vi "Full Force Test SAA.vi"(8 "error in (no error)":errorcluster, 10 "Model in":refnum<class "Model.lvclass">, 11 "Test Actuator State in":refnum<class "Test Actuator State.lvclass">) -> (0 "error out":errorcluster, 1 "Pass":bool, 2 "Model out":refnum<class "Model.lvclass">, 3 "Test Actuator State out":refnum<class "Test Actuator State.lvclass">)   [LabVIEW 2016, in "Test Actuator State.lvclass"]
uses:
  Test Actuator State.lvclass
  Model/Model/Model.lvclass
  Model/Model/Model.lvclass/Model.ctl
  Typedefs/ActuatorSetPoints.ctl
  <vilib>/Platform/TimedLoop/XDataNode/timing_clust.ctl
  <vilib>/Platform/TimedLoop/XDataNode/nitl_modes.ctl
  <vilib>/Platform/TimedLoop/XDataNode/wakeup.ctl
  <vilib>/platform/TimedLoop/XDataNode/XDataNode.xnode
  Typedefs/FAMT Typedefs.lvlib
  <vilib>/Platform/TimedLoop/XDataNode/XDNodeRunTimeDep.lvlib
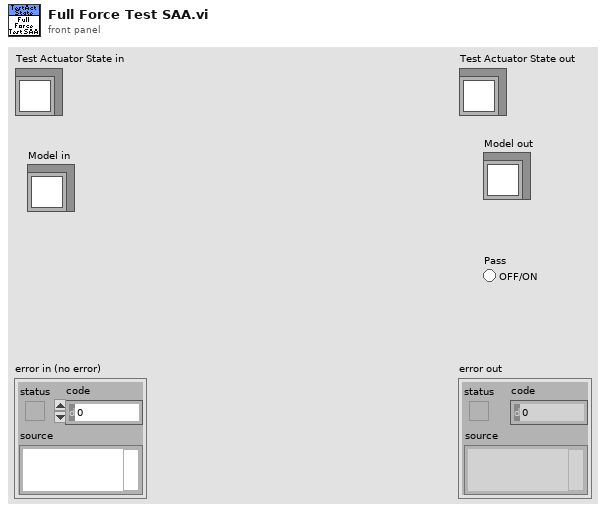
[diagram p1: front panel]
types:
  T1 = typedef "FAMT Typedefs.lvlib/FullForceScanSettings.ctl" = cluster{"Force Tolerance (N)":dbl, "DAA Force Set Points":T2[], "Process Time (s)":dbl, "Sample Time (s)":dbl, "Max Moment (NM)":dbl, "SAA Force Set Points":T2[]}
  T2 = typedef "FAMT Typedefs.lvlib/ForcePair.ctl" = cluster{"Axial Force":dbl, "Lateral Force":dbl}
  T3 = typedef "FAMT Typedefs.lvlib/ActuatorSetPoints.ctl" = cluster{"Axial Force":dbl, "Lateral Force":dbl, "FC1 Force":dbl, "FC2 Force":dbl}
  T4 = typedef "XDNodeRunTimeDep.lvlib/timing_clust.ctl" = cluster{"Expected End [f-1]":u64, "Actual End [f-1]":u64, "Finished Late? [f-1]":bool, "Expected End [i-1]":u64, "Actual End [i-1]":u64, "Finished Late? [i-1]":bool, "Expected Start [i]":u64, "Actual Start [i]":u64, "Expected Start [f]":u64, "Actual Start [f]":u64, "Source Name":string, "Structure Name":string, "Period":i64, "Deadline":i64, "Offset":i64, "Start":i64, "Priority":i32, "Timeout":i32, "Mode":T5, "Wakeup Reason":T6, "Error":errorcluster, "Source Type":string, "Secondary Source Type":string, "Global End Time":u64, "Global Start Time":u64, "Frame Duration":u64, "Iteration Duration":u64, "Assigned CPU":i32, "I/O Scan Engine Mode":u32}
  T5 = typedef "XDNodeRunTimeDep.lvlib/nitl_modes.ctl" = enum32{"No Change", "Process missed periods, maintain original phase", "Discard missed periods, maintain original phase", "Process missed periods, ignore original phase", "Discard missed periods, ignore original phase"}
  T6 = typedef "XDNodeRunTimeDep.lvlib/wakeup.ctl" = enum32{"Normal", "Aborted", "Asynchronous wakeup", "Timing source error", "Timed loop error", "Timeout"}
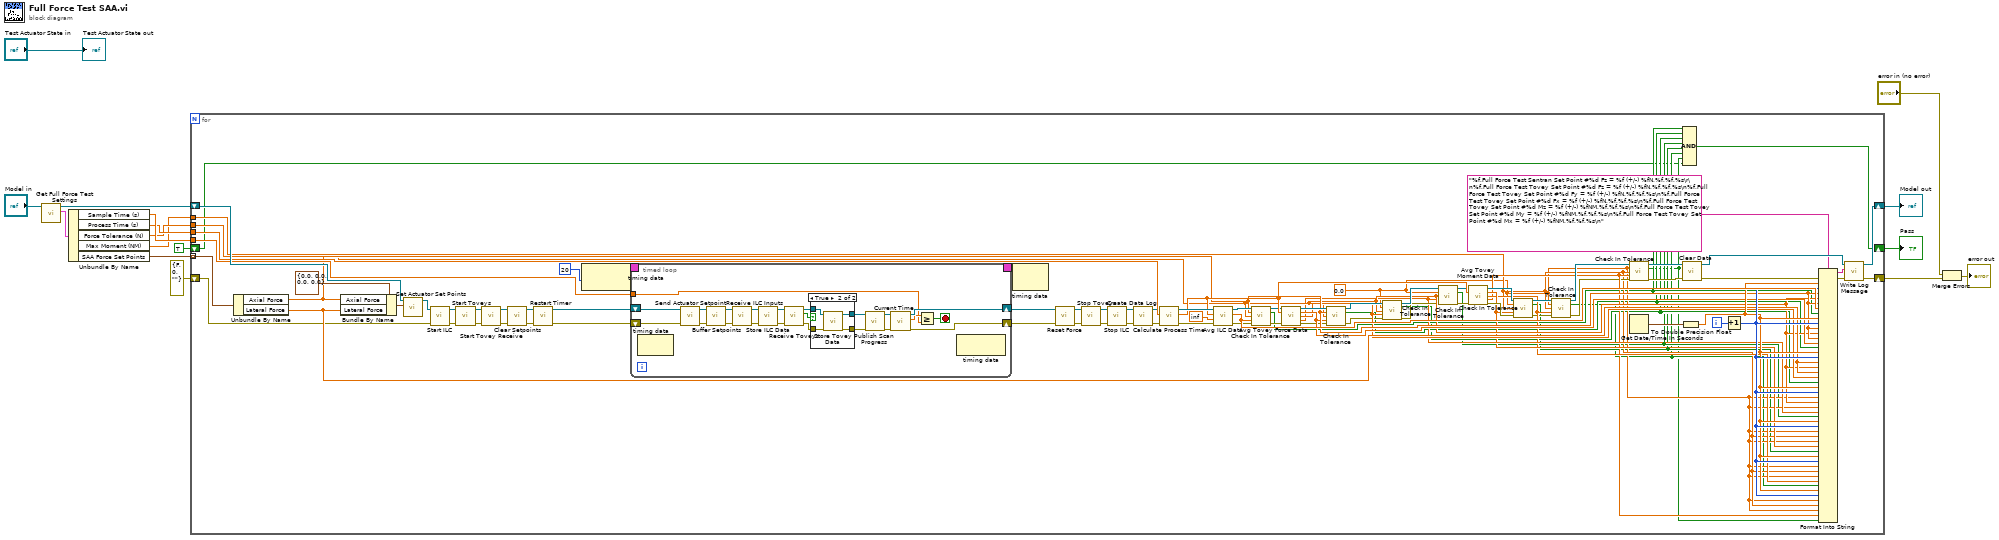
[diagram p0: block diagram]
diagram:
  n1 = call "Get Full Force Test Settings.vi"("Model in"="Model in") -> ("Full Force Test Settings"=w5:T1, "Model out"=w15:refnum<class "Model.lvclass">)  [unwired: 9 in]
  n2 = Unbundle By Name(w5) -> ("Sample Time (s)"=w14:dbl, "Process Time (s)"=w13:dbl, "Force Tolerance (N)"=w12:dbl, "Max Moment (NM)"=w7:dbl, "SAA Force Set Points"=w4:T2[])
  n3 = for {
    tunnel: w4 -> [w94] mode=indexing
    shift-right: [w99] -> w9
    shift-left: w15 -> [w102]
    tunnel: w14 -> [w101]
    tunnel: w13 -> [w89]
    tunnel: w12 -> [w73]
    shift-right: [w90] -> w8
    shift-left: errorcluster {"status"=FALSE, "code"=0, "source"=""} ("error out") -> [w40]
    tunnel: w7 -> [w55]
    shift-right: [w21] -> w1
    shift-left: TRUE -> [w22]
    i -> [w96]
    w54 = 0.0
    n4 = Unbundle By Name(w94) -> ("Axial Force"=w79:dbl, "Lateral Force"=w76:dbl)
    n5 = Bundle By Name(cluster=T3 {"Axial Force"=0.0, "Lateral Force"=0.0, "FC1 Force"=0.0, "FC2 Force"=0.0} ("Actuator Set Points"), "Axial Force"=w79, "Lateral Force"=w76) -> (w95:T3)
    n6 = call "Set Actuator Set Points.vi"("Actuator Set Points"=w95, "Model in"=w102) -> ("Model out"=w41:refnum<class "Model.lvclass">)  [unwired: 9 in]
    n7 = call "Start ILC.vi"("error in (no error)"=w40, "Model in"=w41) -> ("error out"=w39:errorcluster, "Model out"=w38:refnum<class "Model.lvclass">)  [unwired: 8 in]
    n8 = call "Start Toveys.vi"("error in (no error)"=w39, "Model in"=w38) -> ("error out"=w43:errorcluster, "Model out"=w45:refnum<class "Model.lvclass">)  [unwired: 8 in]
    n9 = call "Start Tovey Receive.vi"("error in (no error)"=w43, "Model in"=w45) -> ("error out"=w17:errorcluster, "Model out"=w20:refnum<class "Model.lvclass">)  [unwired: 8 in]
    n10 = call "Clear Setpoints.vi"("error in (no error)"=w17, "Model in"=w20) -> ("error out"=w18:errorcluster, "Model out"=w19:refnum<class "Model.lvclass">)  [unwired: 8 in]
    n11 = call "Restart Timer.vi"("error in (no error)"=w18, "Model in"=w19) -> ("error out"=w42:errorcluster, "Model out"=w44:refnum<class "Model.lvclass">)  [unwired: 8 in]
    n12 = node-c288(i64 20 ("Period")) -> (w50:T4)
    n13 = timed-loop {
      shift-right: [w123] -> w30
      shift-left: w44 -> [w125]
      shift-right: [w122] -> w33
      shift-left: w42 -> [w124]
      tunnel: w101 -> [w120]
      timing: w50 -> [_]
      timing-out: [_] -> w49
      stop <- w119 stop-if-true
      n14 = node-c288() -> ()  [unwired: 1 in, 1 out]
      n15 = call "Send Actuator Setpoint.vi"("error in (no error)"=w124, "Model in"=w125) -> ("error out"=w105:errorcluster, "Model out"=w107:refnum<class "Model.lvclass">)  [unwired: 8 in]
      n16 = call "Buffer Setpoints.vi"("error in (no error)"=w105, "Model in"=w107) -> ("error out"=w104:errorcluster, "Model out"=w106:refnum<class "Model.lvclass">)  [unwired: 8 in]
      n17 = call "Receive ILC Inputs.vi"("error in (no error)"=w104, "Model in"=w106) -> ("error out"=w108:errorcluster, "Model out"=w109:refnum<class "Model.lvclass">)  [unwired: 8 in]
      n18 = call "Store ILC Data.vi"("error in (no error)"=w108, "Model in"=w109) -> ("error out"=w117:errorcluster, "Model out"=w118:refnum<class "Model.lvclass">)  [unwired: 8 in]
      n19 = call "Receive Toveys.vi"("error in (no error)"=w117, "Model in"=w118) -> ("error out"=w115:errorcluster, "Data Received"=w114:bool, "Model out"=w116:refnum<class "Model.lvclass">)  [unwired: 7 in]
      n20 = case shown="True" w114 {
        tunnel: w116 -> [w129 w133]
        tunnel: w115 -> [w128 w132]
        tunnel: [w128 w131] -> w110
        tunnel: [w129 w130] -> w113
        frame False {
        }
        frame True {
          n21 = call "Store Tovey Data.vi"("error in (no error)"=w132, "Model in"=w133) -> ("error out"=w131:errorcluster, "Model out"=w130:refnum<class "Model.lvclass">)  [unwired: 8 in]
        }
      }
      n22 = call "Publish Scan Progress.vi"("error in (no error)"=w110, "Model in"=w113) -> ("error out"=w111:errorcluster, "Model out"=w112:refnum<class "Model.lvclass">)  [unwired: 8 in]
      n23 = call "Current Time.vi"("error in (no error)"=w111, "Model in"=w112) -> ("error out"=w122:errorcluster, "Time"=w121:dbl, "Model out"=w123:refnum<class "Model.lvclass">)  [unwired: 7 in]
      n24 = Greater Or Equal?(x=w121, y=w120) -> (x >= y?=w119:bool)
      n25 = node-c288() -> ()  [unwired: 1 in, 1 out]
    }
    n26 = node-c288(w49) -> ()  [unwired: 1 out]
    n27 = call "Reset Force.vi"("error in (no error)"=w33, "Model in"=w30) -> ("error out"=w32:errorcluster, "Model out"=w31:refnum<class "Model.lvclass">)  [unwired: 8 in]
    n28 = call "Stop Toveys.vi"("error in (no error)"=w32, "Model in"=w31) -> ("error out"=w37:errorcluster, "Model out"=w36:refnum<class "Model.lvclass">)  [unwired: 8 in]
    n29 = call "Stop ILC.vi"("error in (no error)"=w37, "Model in"=w36) -> ("error out"=w34:errorcluster, "Model out"=w35:refnum<class "Model.lvclass">)  [unwired: 8 in]
    n30 = call "Create Data Log.vi"("error in (no error)"=w34, "Model in"=w35) -> ("error out"=w46:errorcluster, "Model out"=w47:refnum<class "Model.lvclass">)  [unwired: 8 in]
    n31 = call "Calculate Process Time.vi"("error in (no error)"=w46, "Seconds"=w89, "Model in"=w47) -> ("error out"=w87:errorcluster, "Time"=w86:dbl, "Model out"=w88:refnum<class "Model.lvclass">)  [unwired: 6 in]
    n32 = call "Avg ILC Data.vi"("error in (no error)"=w87, "Before This Time"=inf, "After This Time"=w86, "Model in"=w88) -> ("error out"=w83:errorcluster, "Fz"=w84:dbl, "Model out"=w85:refnum<class "Model.lvclass">)  [unwired: 4 in, 1 out]
    n33 = call "Check In Tolerance.vi"("Model in"=w85, "Expected"=w79, "Tolerance"=w73, "Actual"=w84, "error in (no error)"=w83) -> ("Model out"=w53:refnum<class "Model.lvclass">, "Pass"=w29:bool, "error out"=w52:errorcluster)  [unwired: 8 in]
    n34 = call "Avg Tovey Force Data.vi"("Model in"=w53, "After This Time"=w86, "error in (no error)"=w52) -> ("Model out"=w80:refnum<class "Model.lvclass">, "Fz"=w78:dbl, "Fy"=w75:dbl, "Fx"=w65:dbl, "error out"=w72:errorcluster)  [unwired: 8 in]
    n35 = call "Check In Tolerance.vi"("Model in"=w80, "Expected"=w79, "Tolerance"=w73, "Actual"=w78, "error in (no error)"=w72) -> ("Model out"=w77:refnum<class "Model.lvclass">, "Pass"=w28:bool, "error out"=w71:errorcluster)  [unwired: 8 in]
    n36 = call "Check In Tolerance.vi"("Model in"=w77, "Expected"=w54, "Tolerance"=w73, "Actual"=w75, "error in (no error)"=w71) -> ("Model out"=w74:refnum<class "Model.lvclass">, "Pass"=w27:bool, "error out"=w70:errorcluster)  [unwired: 8 in]
    n37 = call "Check In Tolerance.vi"("Model in"=w74, "Expected"=w54, "Tolerance"=w73, "Actual"=w65, "error in (no error)"=w70) -> ("Model out"=w68:refnum<class "Model.lvclass">, "Pass"=w26:bool, "error out"=w69:errorcluster)  [unwired: 8 in]
    n38 = call "Avg Tovey Moment Data.vi"("Model in"=w68, "After This Time"=w86, "error in (no error)"=w69) -> ("Model out"=w67:refnum<class "Model.lvclass">, "Mz"=w64:dbl, "My"=w61:dbl, "Mx"=w60:dbl, "error out"=w66:errorcluster)  [unwired: 8 in]
    n39 = call "Check In Tolerance.vi"("Model in"=w67, "Expected"=w54, "Tolerance"=w55, "Actual"=w64, "error in (no error)"=w66) -> ("Model out"=w63:refnum<class "Model.lvclass">, "Pass"=w25:bool, "error out"=w58:errorcluster)  [unwired: 8 in]
    n40 = call "Check In Tolerance.vi"("Model in"=w63, "Expected"=w54, "Tolerance"=w55, "Actual"=w61, "error in (no error)"=w58) -> ("Model out"=w62:refnum<class "Model.lvclass">, "Pass"=w24:bool, "error out"=w57:errorcluster)  [unwired: 8 in]
    n41 = call "Check In Tolerance.vi"("Model in"=w62, "Expected"=w54, "Tolerance"=w55, "Actual"=w60, "error in (no error)"=w57) -> ("Model out"=w59:refnum<class "Model.lvclass">, "Pass"=w23:bool, "error out"=w56:errorcluster)  [unwired: 8 in]
    n42 = Get Date/Time In Seconds() -> (seconds since 1Jan1904=w97:timestamp)
    n43 = To Double Precision Float(number=w97) -> (double precision float=w81:dbl)
    n44 = call "Clear Data.vi"("error in (no error)"=w56, "Model in"=w59) -> ("error out"=w92:errorcluster, "Model out"=w100:refnum<class "Model.lvclass">)  [unwired: 8 in]
    n45 = Compound Arithmetic op=AND(w29, w28, w27, w26, w25, w24, w23, w22) -> (w21:bool)
    n46 = Increment(x=w96) -> (x+1=w82:i32)
    n47 = Format Into String(format string="%f,Full Force Test Sentran Set Point #%d Fz = %f (+/-) %fN,%f,%f,%s\r\n%f,Full Force Test Tovey Set Point #%d Fz = %f (+/-) %fN,%f,%f,%s\n%f,Full Force Test Tovey Set Point #%d Fy = %f (+/-) %fN,%f,%f,%s\n%f,Full Force Test Tovey Set Point #%d Fx = %f (+/-) %fN,%f,%f,%s\n%f,Full Force Test Tovey Set Point #%d Mz = %f (+/-) %fNM,%f,%f,%s\n%f,Full Force Test Tovey Set Point #%d My = %f (+/-) %fNM,%f,%f,%s\n%f,Full Force Test Tovey Set Point #%d Mx = %f (+/-) %fNM,%f,%f,%s\n", error in=w92, w81, w82, w79, w73, w79, w84, w29, w81, w82, w79, w73, w79, w78, w28, w81, w82, w76, w73, w76, w75, w27, w81, w82, w54, w73, w54, w65, w26, w81, w82, w54, w55, w54, w64, w25, w81, w82, w54, w55, w54, w61, w24, w81, w82, w54, w55, w54, w60, w23) -> (resulting string=w93:string, error out=w91:errorcluster)  [unwired: 1 in]
    n48 = call "Write Log Message.vi"("error in (no error)"=w91, "Message"=w93, "Model in"=w100) -> ("error out"=w90:errorcluster, "Model out"=w99:refnum<class "Model.lvclass">)  [unwired: 7 in]
  }
  "Model out" <- w9
  "Pass" <- w1
  n49 = Merge Errors("error in (no error)", w8) -> (→"error out":errorcluster)
  "Test Actuator State out" <- "Test Actuator State in"
